vi "editscenario Query DB for Scenario.vi"(8 "error in (no error)":errorcluster, 10 "sxScenarioId (\"\")":string, 11 "Connection Refnum":T1) -> (0 "error out":errorcluster, 2 "Scenario Record":T2, 3 "Connection Refnum":T1)   [LabVIEW 2011]
uses:
  server/database/Scenarios/Scenario Record.ctl
  server/database/Scenarios/Conditions/Condition Record.ctl
  server/database/Scenarios/Conditions/Condition Operators.ctl
  Summitek EXT/ODBC/SQL Controls/Connection Refnum.ctl
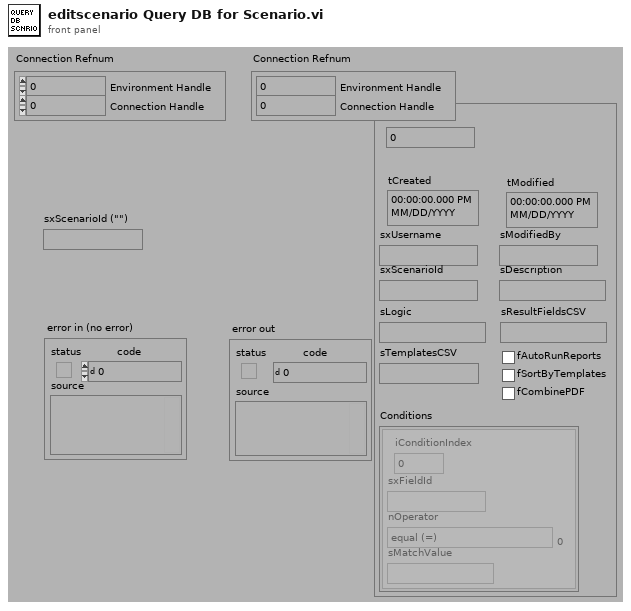
[diagram p1: front panel]
types:
  T1 = typedef "Connection Refnum.ctl" = cluster{"Environment Handle":i32, "Connection Handle":i32}
  T2 = typedef "Scenario Record.ctl" = cluster{"ixScenario":i32, "tCreated":timestamp, "tModified":timestamp, "sxUsername":string, "sModifiedBy":string, "sxScenarioId":string, "sDescription":string, "sLogic":string, "sResultFieldsCSV":string, "sTemplatesCSV":string, "fAutoRunReports":bool, "fSortByTemplates":bool, "fCombinePDF":bool, "Conditions":T3[]}
  T3 = typedef "Condition Record.ctl" = cluster{"iConditionIndex":i32, "sxFieldId":string, "nOperator":T4, "sMatchValue":string}
  T4 = typedef "Condition Operators.ctl" = enum16{"equal (=)", "not equal (\\u2260)", "less than (<)", "less than or equal (\\u2264)", "greater than (>)", "greater than or equal (\\u2265)", "contains", "does not contain"}
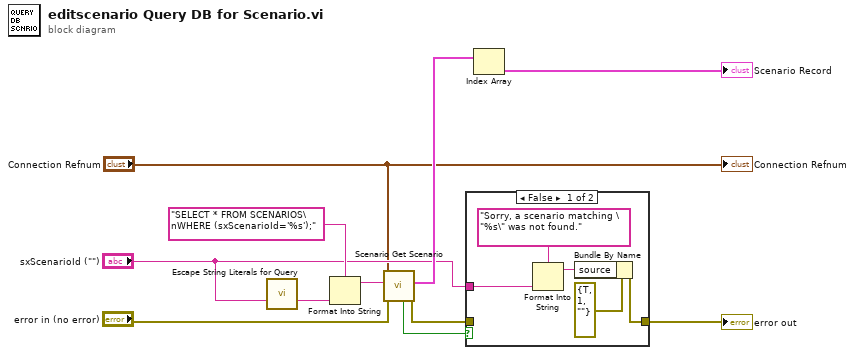
[diagram p0: block diagram]
diagram:
  n1 = call "Escape String Literals for Query.vi"("String"="sxScenarioId (\"\")") -> ("escaped String"=w1:string)  [unwired: 1 in, 13 out]
  n2 = Format Into String(format string="SELECT * FROM SCENARIOS\nWHERE (sxScenarioId='%s');", w1) -> (resulting string=w2:string)  [unwired: 2 in, 1 out]
  n3 = call "Scenario Get Scenario.vi"("error in (no error)"="error in (no error)", "Query"=w2, "Connection Refnum"="Connection Refnum") -> ("error out"=w9:errorcluster, "Scenarios"=w8:T2[], "Data Present?"=w10:bool)  [unwired: 6 out]
  n4 = case shown="False" w10 {
    tunnel: w9 -> [_ w17]
    tunnel: [w13 w17] -> w5
    tunnel: "sxScenarioId (\"\")" -> [w12 _]
    frame False {
      n5 = Format Into String(format string="Sorry, a scenario matching \"%s\" was not found.", w12) -> (resulting string=w15:string)  [unwired: 2 in, 1 out]
      n6 = Bundle By Name(cluster=errorcluster {"status"=TRUE, "code"=1, "source"=""} ("error out"), "source"=w15) -> (w13:errorcluster)
    }
    frame True {
    }
  }
  "error out" <- w5
  n7 = Index Array(array=w8) -> (element=→"Scenario Record":T2)  [unwired: 1 in]
  "Connection Refnum" <- "Connection Refnum"
